vi "Initialize Interface.vi"(8 "error in (no error)":errorcluster, 10 "interface":string, 11 "PXImc Transceiver in":refnum<class "PXImc Transceiver.lvclass">) -> (0 "error out":errorcluster, 3 "PXImc Transceiver out":refnum<class "PXImc Transceiver.lvclass">)   [LabVIEW 2017, in "PXImc.lvlib" / "PXImc Transceiver.lvclass"]
uses:
  PXImc Transceiver.lvclass
  PXImc Transceiver.lvclass/PXImc Transceiver.ctl
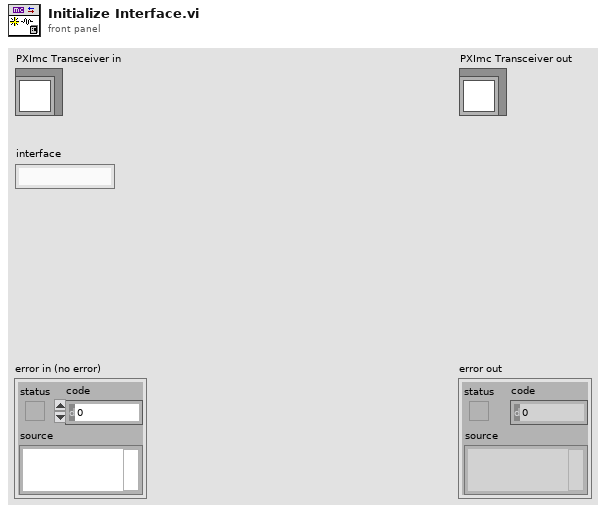
[diagram p1: front panel]
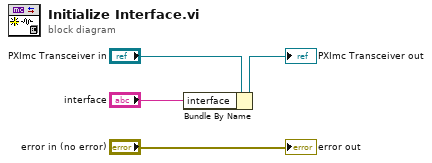
[diagram p0: block diagram]
diagram:
  n1 = Bundle By Name(cluster="PXImc Transceiver in", "interface"="interface") -> (→"PXImc Transceiver out":refnum<class "PXImc Transceiver.lvclass">)
  "error out" <- "error in (no error)"
